vi "Number bracket comparator.vi"(8 "Min Number":dbl, 10 "Actual Number":dbl, 11 "Max Number":dbl) -> (1 "Below Min":bool, 2 "Above Max":bool)   [LabVIEW 2011]
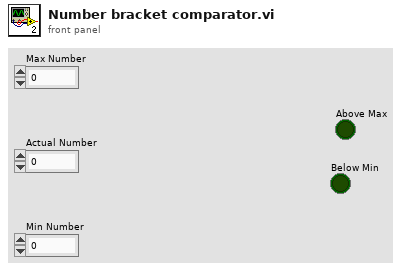
[diagram p1: front panel]
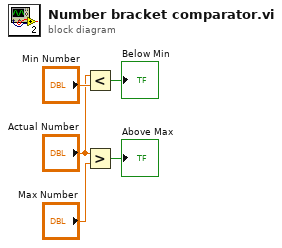
[diagram p0: block diagram]
diagram:
  n1 = Less?(x="Actual Number", y="Min Number") -> (x < y?=→"Below Min":bool)
  n2 = Greater?(x="Actual Number", y="Max Number") -> (0:→"Above Max":bool)
